vi "Running Average Settings.vi"(8 "error in (no error)":errorcluster, 11 "Node Ptr":T1 format="%.0x") -> (0 "error out":errorcluster)   [LabVIEW 2017, in "Waveform-Processing-Custom-Device System Explorer.lvlib"]
uses:
  Waveform-Processing-Custom-Device System Explorer.lvlib
  <vilib>/NI Veristand/Custom Device API/Custom Device Item Ref.ctl
  <vilib>/NI VeriStand/Custom Device API/Custom Device API.lvlib
panel:
  in  "SHDocVw.IWebBrowser":refnum<k7>(container)
  in  "Specific Header":cluster{"Section Name":string}={"Section Name"="Specific Page Settings"}
  in  "General Header":cluster{"Section Name":string}={"Section Name"="General Page Settings"}
  in  "Description":string
  in  "Name":string
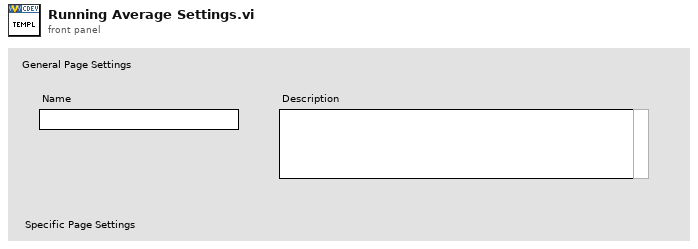
[diagram p1: front panel]
types:
  T1 = typedef "Custom Device API.lvlib/Custom Device Item Ref.ctl" = u64
  T2 = typedef "Custom Device API.lvlib/Custom Device Item Info.ctl" = cluster{"Name":string, "Is Channel":bool, "GUID":string, "Is Waveform":bool}
  T3 = typedef "Custom Device API.lvlib/Custom Device Commands.ctl" = enum16{"Default", "Item renamed", "Shutdown", "Dynamic button pressed"}
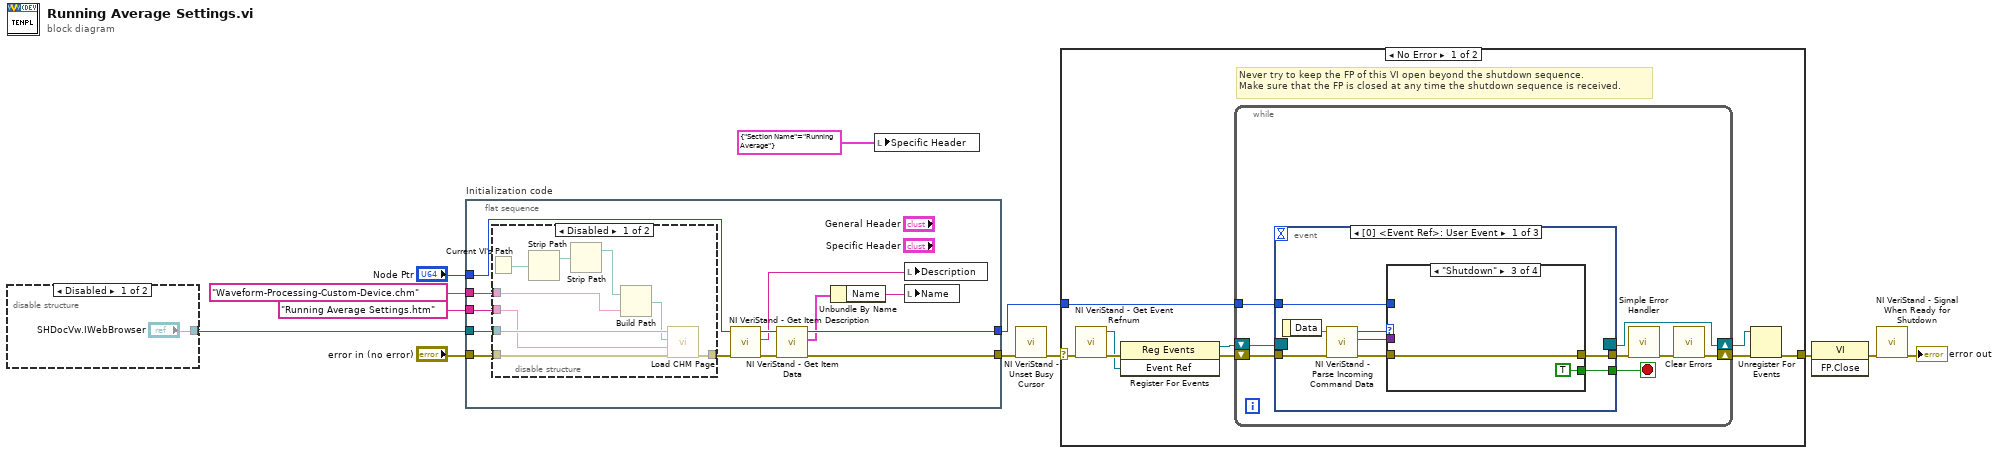
[diagram p0: block diagram]
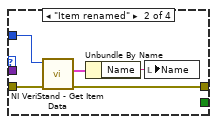
[diagram p4: hidden frame]
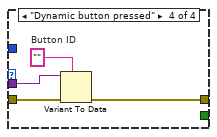
[diagram p5: hidden frame]
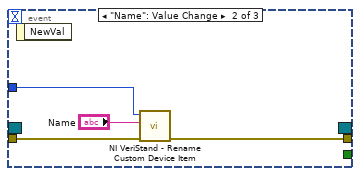
[diagram p6: hidden frame]
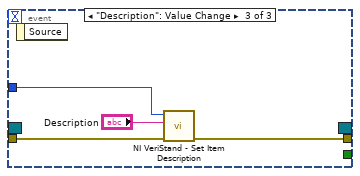
[diagram p7: hidden frame]
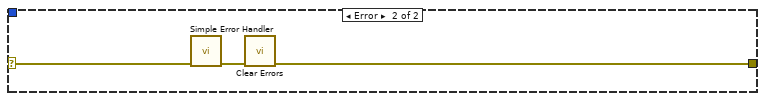
[diagram p8: hidden frame]
diagram:
  n1 = disable-structure shown="Disabled" {
    disable-tunnel: ["SHDocVw.IWebBrowser" _] -> w2
    frame Disabled {
    }
    frame Enabled {
    }
  }
  n2 = flat-sequence "Initialization code" {
    tunnel: "error in (no error)" -> [w16]
    tunnel: "Node Ptr" -> [w14]
    tunnel: [w22] -> w8
    tunnel: [w26] -> w5
    tunnel: "Running Average Settings.htm" ("CD_CHM_Section") -> [w18]
    tunnel: "Waveform-Processing-Custom-Device.chm" ("CD_CHM_FileName") -> [w19]
    tunnel: w2 -> [w17]
    frame #0 {
      n3 = disable-structure shown="Disabled" {
        disable-tunnel: w16 -> [w35 w36]
        disable-tunnel: [w34 w36] -> w15
        disable-tunnel: w17 -> [w33 _]
        disable-tunnel: w18 -> [w32 _]
        disable-tunnel: w19 -> [w28 _]
        frame Disabled {
          n4 = Current VI's Path() -> (path=w31:path)
          n5 = Strip Path(path=w31) -> (stripped path=w30:path)  [unwired: 1 out]
          n6 = Strip Path(path=w30) -> (stripped path=w29:path)  [unwired: 1 out]
          n7 = Build Path(base path=w29, name or relative path=w28) -> (appended path=w27:path)
          n8 = call <vilib>:"Load CHM Page.vi"("error in (no error)"=w35, "HTML File"=w32, "Compiled CHM Path"=w27, "Web Browser Reference"=w33) -> ("error out"=w34:errorcluster)  [unwired: 7 in]
        }
        frame Enabled {
        }
      }
      n9 = call <vilib>:"NI VeriStand - Get Item Description.vi"("error in (no error)"=w15, "Item Ref in"=w14) -> ("error out"=w24:errorcluster, "Description"=w20:string, "Item Ref out"=w25:T1)  [unwired: 7 out]
      n10 = call <vilib>:"NI VeriStand - Get Item Data.vi"("error in (no error)"=w24, "Item Ref in"=w25) -> ("error out"=w22:errorcluster, "Item Info"=w23:T2, "Item Ref out"=w26:T1)  [unwired: 7 out]
      n11 = Unbundle By Name(w23) -> ("Name"=w21:string)
      n12 = local write "Description"(w20) -> ()
      n13 = local write "Name"(w21) -> ()
    }
  }
  n14 = local write "Specific Header"(cluster{"Section Name":string} {"Section Name"="Running Average"} ("Specific Header")) -> ()
  n15 = call <vilib>:"NI VeriStand - Unset Busy Cursor.vi"("error in (no error)"=w8) -> ("error out"=w7:errorcluster)  [unwired: 10 out]
  n16 = case shown="No Error" w7 {
    selector: w7 -> [w37 w84]
    tunnel: [w42 w82] -> w12
    tunnel: w5 -> [w38 _]
    frame No Error {
      # "Never try to keep the FP of this VI open beyond the shutdown sequence.\nMake sure that the FP is closed at any time the shutdown sequence is received."
      n17 = call <vilib>:"NI VeriStand - Get Event Refnum.vi"("error in (no error)"=w37) -> ("error out"=w45:errorcluster, "Event Ref"=w41:refnum<user-event>)  [unwired: 9 out]
      n18 = register-events(error in=w45, w41) -> (reference out=w39:refnum<event-registration>, error out=w40:errorcluster)  [unwired: 1 in]
      n19 = while {
        tunnel: w38 -> [w49]
        shift-right: [w46] -> w43
        shift-left: w40 -> [w52]
        shift-right: [w53] -> w44
        shift-left: w39 -> [w51]
        stop <- w50 stop-if-true
        n20 = event shown="[0] <Event Ref>: User Event" {
          selector: w51 -> [_ _ _]
          dyn-events: [_ _ _] -> w53
          timeout: _ -> [_ _ _]
          tunnel: w52 -> [w61 w77 w80]
          tunnel: [w57 _ _] -> w50
          tunnel: [w56 w76 w79] -> w48
          tunnel: w49 -> [w55 w75 w81]
          event User Event {
            n21 = event-data() -> ("Data"=w60:string)  [unwired: 1 out]
            n22 = call <vilib>:"NI VeriStand - Parse Incoming Command Data.vi"("error in (no error)"=w61, "Incoming data"=w60) -> ("error out"=w59:errorcluster, "Outgoing data"=w54:variant, "Action"=w58:T3)  [unwired: 7 out]
            n23 = case shown="\"Shutdown\"" w58 {
              tunnel: w59 -> [w62 w67 w68 w73]
              tunnel: [_ _ TRUE _] -> w57
              tunnel: [w62 w64 w68 w70] -> w56
              tunnel: w55 -> [_ w66 _ _]
              tunnel: w54 -> [_ _ _ w72]
              frame "Default", Default {
              }
              frame "Item renamed" {
                n24 = call <vilib>:"NI VeriStand - Get Item Data.vi"("error in (no error)"=w67, "Item Ref in"=w66) -> ("error out"=w64:errorcluster, "Item Info"=w65:T2)  [unwired: 8 out]
                n25 = Unbundle By Name(w65) -> ("Name"=w63:string)
                n26 = local write "Name"(w63) -> ()
              }
              frame "Shutdown" {
              }
              frame "Dynamic button pressed" {
                w71 = ""  # Button ID
                n27 = Variant To Data(error in=w73, type=w71, Variant=w72) -> (error out=w70:errorcluster)  [unwired: 1 out]
              }
            }
          }
          event "Name": Value Change {
            n28 = event-data() -> ()  [unwired: 2 out]
            n29 = call <vilib>:"NI VeriStand - Rename Custom Device Item.vi"("error in (no error)"=w77, "New Name"="Name", "Item Ref in"=w75) -> ("error out"=w76:errorcluster)  [unwired: 1 in, 7 out]
          }
          event "Description": Value Change {
            n30 = event-data() -> ()  [unwired: 2 out]
            n31 = call <vilib>:"NI VeriStand - Set Item Description.vi"("error in (no error)"=w80, "Description"="Description", "Item Ref in"=w81) -> ("error out"=w79:errorcluster)  [unwired: 8 out]
          }
        }
        n32 = call <vilib>:"Simple Error Handler.vi"("error in (no error)"=w48) -> ("error out"=w47:errorcluster)  [unwired: 1 in, 7 out]
        n33 = call <vilib>:"Clear Errors.vi"("error in (no error)"=w47) -> ("error out"=w46:errorcluster)  [unwired: 1 in, 5 out]
      }
      n34 = Unregister For Events(event registration refnum=w44, error in=w43) -> (error out=w42:errorcluster)
    }
    frame Error {
      n35 = call <vilib>:"Simple Error Handler.vi"("error in (no error)"=w84) -> ("error out"=w83:errorcluster)  [unwired: 1 in, 7 out]
      n36 = call <vilib>:"Clear Errors.vi"("error in (no error)"=w83) -> ("error out"=w82:errorcluster)  [unwired: 1 in, 5 out]
    }
  }
  n37 = invoke class="VI" method="FP.Close"(error in=w12) -> (error out=w11:errorcluster)  [unwired: 2 in, 2 out]
  n38 = call <vilib>:"NI VeriStand - Signal When Ready for Shutdown.vi"("error in (no error)"=w11) -> ("error out"=→"error out":errorcluster)  [unwired: 10 out]
